vi "destroy Server.vi"(8 "error in (no error)":errorcluster, 11 "pServerId":i32) -> (0 "error out":errorcluster, 3 "function return":i32)   [LabVIEW 2012, in "clearvolume.lvlib"]
doc: "__declspec(dllexport) long __cdecl destroyServer( long pServerId);"
uses:
  clearvolume.lvlib
  clearvolume.dll
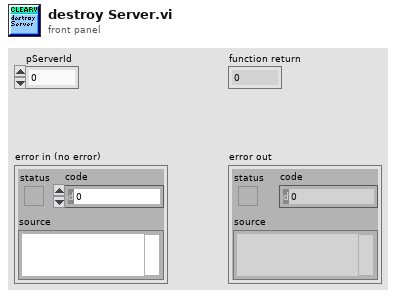
[diagram p1: front panel]
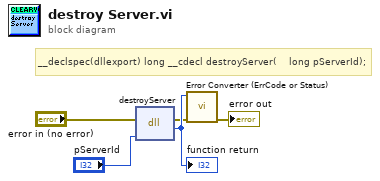
[diagram p0: block diagram]
diagram:
  # "__declspec(dllexport) long __cdecl destroyServer(\t\t\t\tlong pServerId);"
  n1 = dll-call lib="C:/Users/myerslab/workspace/Libraries/CV/clearvolume/src/labview/clearvolume/clearvolume.*" fn="destroyServer"(error in="error in (no error)", "pServerId"="pServerId") -> (error out=w2:errorcluster, w5:i32)  [unwired: 3 in, 1 out]
  "function return" <- w5
  n2 = call "Error Converter (ErrCode or Status).vi"("error in (no error)"=w2, "error code"=w5) -> ("error out"=→"error out":errorcluster)  [unwired: 9 in]
